vi "mono_camera_test.vi"() -> ()   [LabVIEW 2018]
panel:
  out "camera_out":picture
  in  "stop":bool
  in  "streeing_angle":dbl(knob) scale=-1.0..1.0
  in  "throttle":dbl(slide) scale=-1.0..1.0
  out "Speed":dbl(knob) scale=0.0..200.0
  out "monodrive_python":path=path "C:/Users/celit/Documents/GitHub/client/lv_test.py"
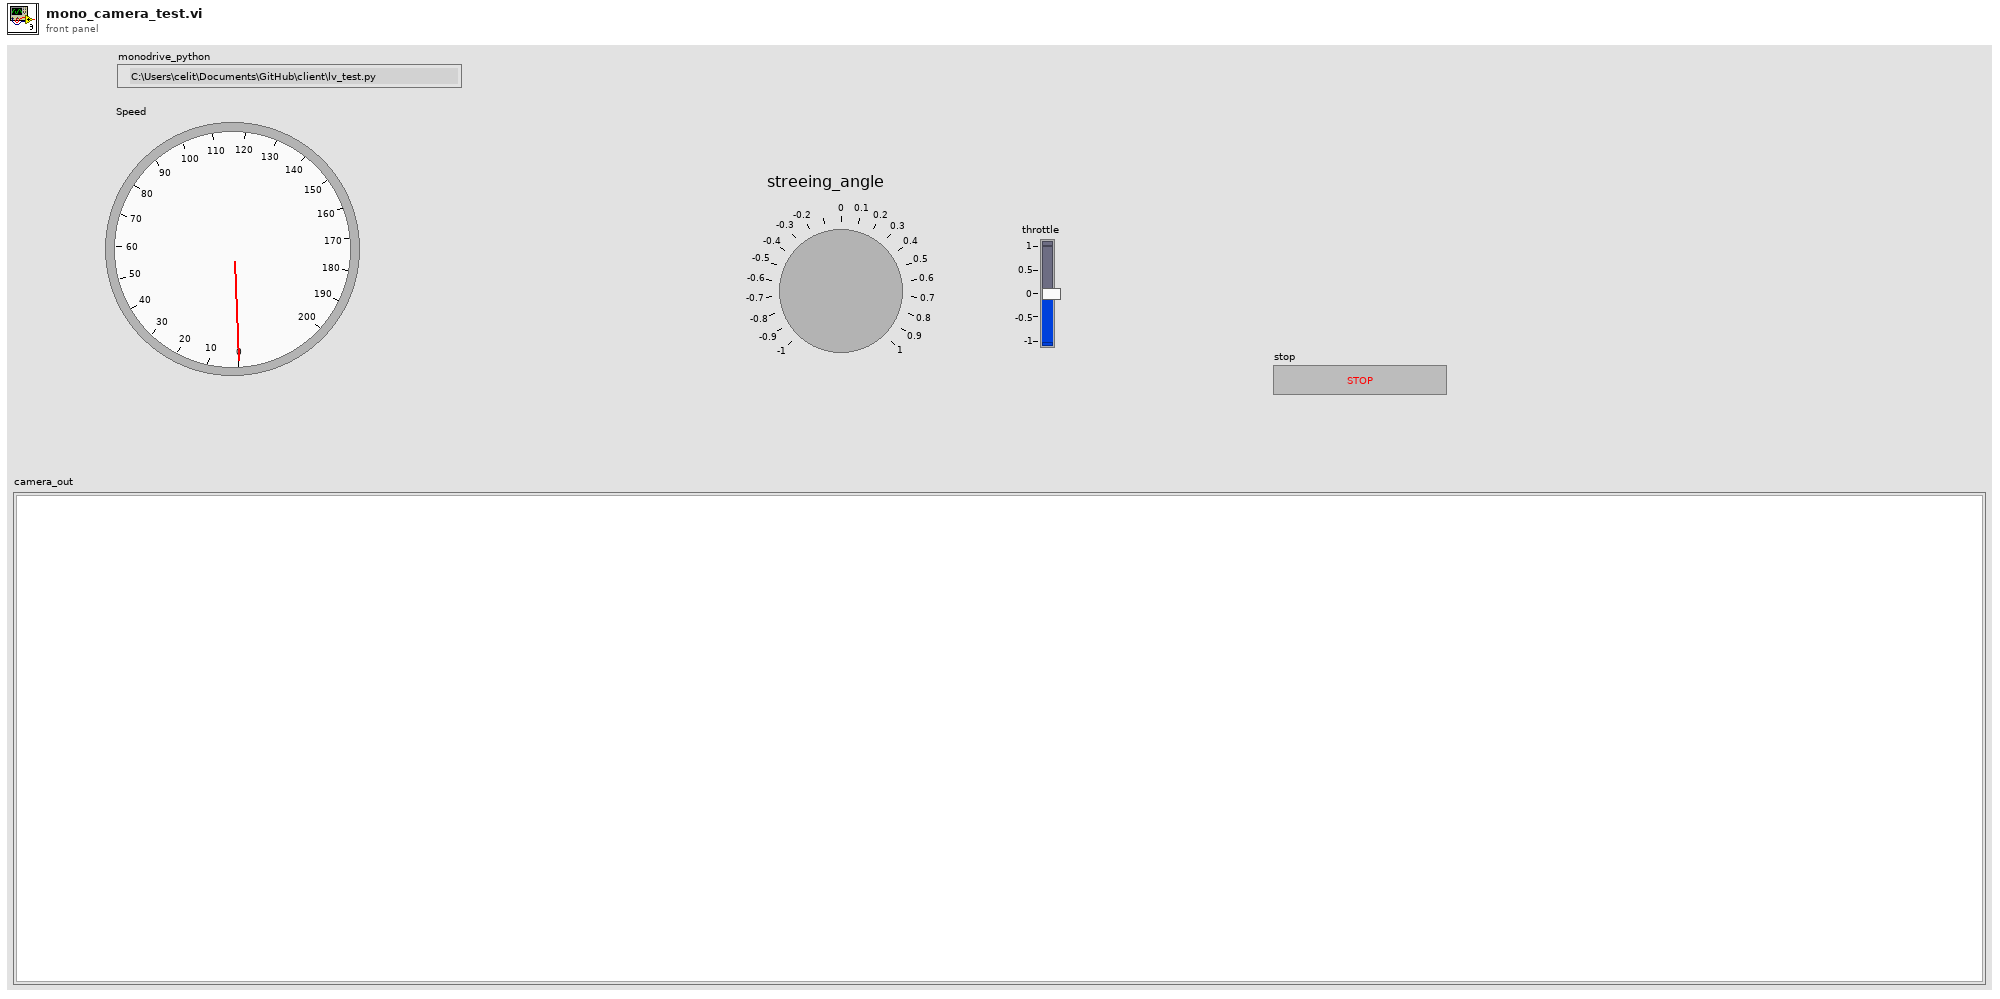
[diagram p1: front panel]
types:
  T1 = cluster{"sensor":string, "address":string, "remote port or service name":u16}
  T2 = cluster{"sensor":string, "connection ID":refnum<k5>, "error out":errorcluster}
  T3 = cluster{cluster{"length":u32, "time_stamp":u32, "game_time":sgl}, "data out":string}
  T4 = typedef "imagedata.ctl" = cluster{"image type":i32, "image depth":i32, "image":u8[], "mask":u8[], "colors":u32[], "Rectangle":cluster{"left":i16, "top":i16, "right":i16, "bottom":i16}}
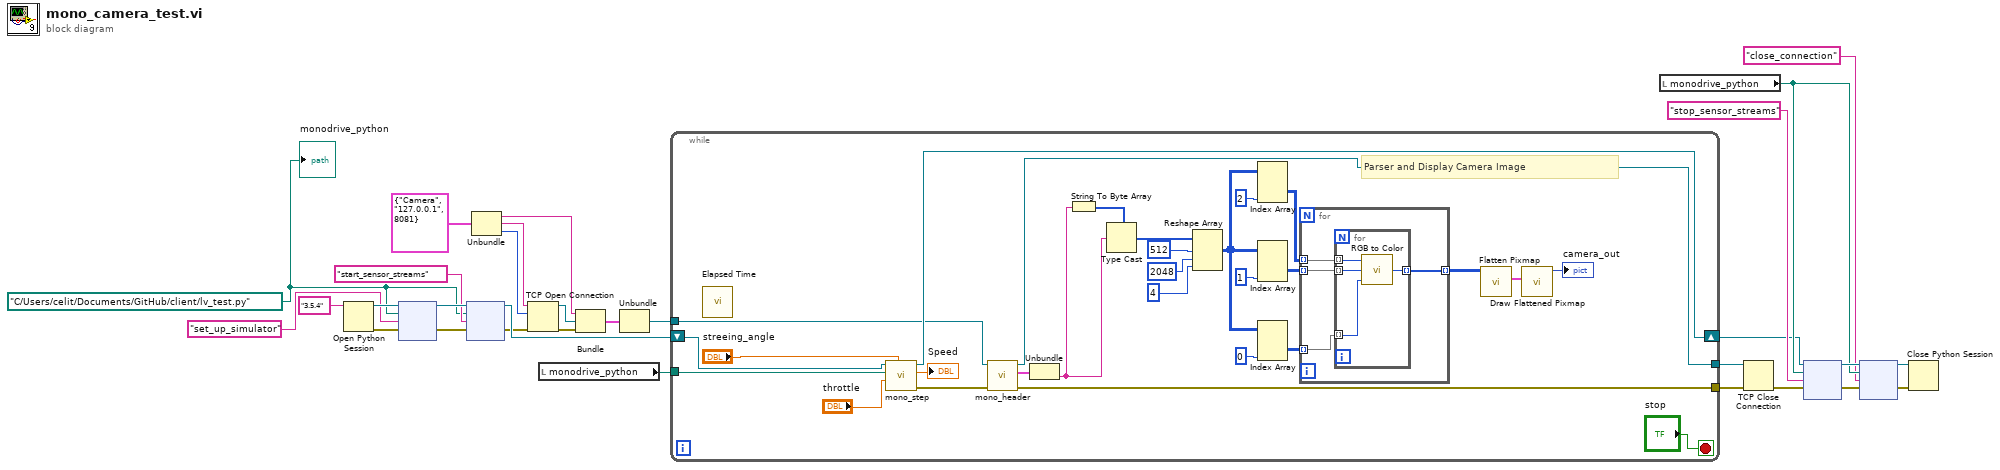
[diagram p0: block diagram]
diagram:
  w23 = path "C:/Users/celit/Documents/GitHub/client/lv_test.py" ("Python Module Path")
  n1 = Open Python Session(python version="3.5.4" ("Python version")) -> (session out=w27:refnum<k35>, error out=w28:errorcluster)  [unwired: 2 in]
  n2 = node(w27, w23, "set_up_simulator" ("function name"), w28) -> (w29:refnum<k35>, w30:errorcluster)  [unwired: 2 in, 2 out]
  n3 = node(w29, w23, "start_sensor_streams" ("function name"), w30) -> (w11:refnum<k35>, w2:errorcluster)  [unwired: 2 in, 2 out]
  n4 = Unbundle(T1 {"sensor"="Camera", "address"="127.0.0.1", "remote port or service name"=8081} ("Cluster in")) -> ("sensor"=w6:string, "address"=w4:string, "remote port or service name"=w5:u16)
  n5 = TCP Open Connection(address=w4, remote port or service name=w5, error in (no error)=w2) -> (connection ID=w7:refnum<k5>, error out=w8:errorcluster)  [unwired: 2 in]
  n6 = local read "monodrive_python"() -> (w12:path)
  n7 = Bundle("sensor"=w6, "connection ID"=w7, "error out"=w8) -> (w9:T2)  [unwired: 1 in]
  n8 = Unbundle(w9) -> ("connection ID"=w1:refnum<k5>)  [unwired: 2 out]
  n9 = while {
    tunnel: [w53] -> w22
    tunnel: [w52] -> w21
    tunnel: w12 -> [w49]
    shift-right: [w48] -> w10
    shift-left: w11 -> [w51]
    tunnel: w1 -> [w45]
    stop <- "stop" stop-if-true
    # "Parser and Display Camera Image"
    n10 = call "Elapsed Time"() -> ()  [unwired: 12 in, 8 out]
    n11 = call "mono_step.vi"("Steering Wheel Angle"="streeing_angle", "Throttle"="throttle", "Python Module Path"=w49, "Refnum in"=w51) -> ("error_out"=w55:errorcluster, "Speed"=→"Speed":dbl, "Refnum out"=w48:refnum<k35>)  [unwired: 4 in, 1 out]
    n12 = call "mono_header.vi"("error in"=w55, "connection ID"=w45) -> ("error out"=w53:errorcluster, "sensor_sample"=w54:T3, "connection ID out"=w52:refnum<k5>)  [unwired: 7 in]
    n13 = Unbundle(w54) -> ("data out"=w57:string)  [unwired: 1 out]
    n14 = String To Byte Array(string=w57) -> (unsigned byte array=w58:u8[])
    n15 = Type Cast(type=w58, x=w57) -> (*(type *) &x=w40:u8[])
    n16 = Reshape Array(w40, 512 ("dimension size"), 2048 ("dimension size"), 4 ("dimension size")) -> (w37:u8[][][])
    n17 = Index Array(array=w37, index (dim 2)=2 ("index (col)")) -> (element=w36:u8[][])  [unwired: 2 in]
    n18 = Index Array(array=w37, index (dim 2)=1 ("index (col)")) -> (element=w35:u8[][])  [unwired: 2 in]
    n19 = Index Array(array=w37, index (dim 2)=0 ("disabled index (col)")) -> (element=w34:u8[][])  [unwired: 2 in]
    n20 = for {
      tunnel: w36 -> [w62] mode=indexing
      tunnel: w35 -> [w61] mode=indexing
      tunnel: w34 -> [w60] mode=indexing
      tunnel: [w59] -> w33 mode=indexing
      n21 = for {
        tunnel: w62 -> [w66] mode=indexing
        tunnel: w61 -> [w65] mode=indexing
        tunnel: w60 -> [w64] mode=indexing
        tunnel: [w63] -> w59 mode=indexing
        n22 = call <vilib>:"RGB to Color.vi"("B"=w64, "G"=w65, "R"=w66) -> ("Color"=w63:u32)
      }
    }
    n23 = call <vilib>:"Flatten Pixmap.vi"("24-bit pixmap"=w33) -> ("image data"=w32:T4)  [unwired: 10 in]
    n24 = call <vilib>:"Draw Flattened Pixmap.vi"("image data"=w32) -> ("new picture"=→"camera_out":picture)  [unwired: 8 in]
  }
  n25 = local read "monodrive_python"() -> (w15:path)
  n26 = TCP Close Connection(connection ID=w21, error in (no error)=w22) -> (error out=w14:errorcluster)  [unwired: 1 in, 1 out]
  n27 = node(w10, w15, "stop_sensor_streams" ("function name"), w14) -> (w20:refnum<k35>, w19:errorcluster)  [unwired: 2 in, 2 out]
  n28 = node(w20, w15, "close_connection" ("function name"), w19) -> (w18:refnum<k35>, w17:errorcluster)  [unwired: 2 in, 2 out]
  n29 = Close Python Session(session in=w18, error in=w17) -> ()  [unwired: 1 out]
  "monodrive_python" <- w23
